vi "Test_ADC.vi"() -> ()   [LabVIEW 2012]
uses:
  STM32-CoreBD.lvlib
panel:
  out "Error":u32
  out "Error Out":errorcluster caption="错误输出"
  in  "停止":bool
  out "数值":i32
  out "波形图":waveform(dbl)(graph)
  in  "SampleRate":u32=250000 min=1000 max=250000 step=1000
  in  "Points(X*5k)":u8=1 min=1 max=100
  in  "Channel":enum16{"Channel A", "Channel B"}(ring)
  in  "VISA资源输入":refnum<visa-resource-name>
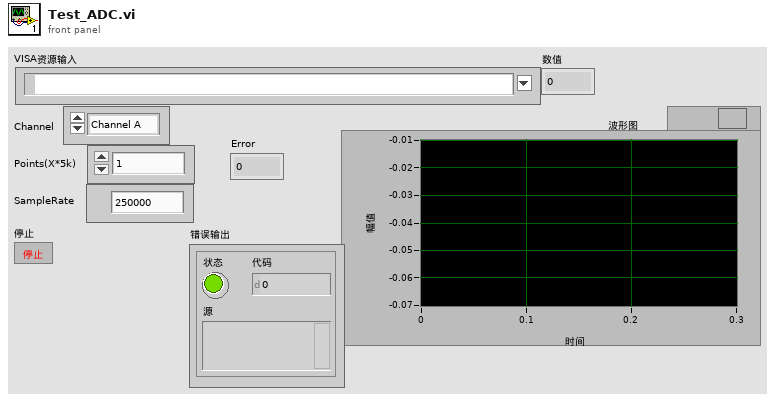
[diagram p1: front panel]
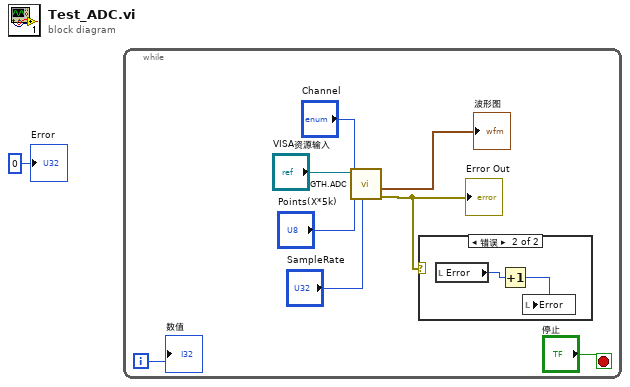
[diagram p0: block diagram]
diagram:
  n1 = while {
    i -> [w4]
    stop <- "停止" stop-if-true
    n2 = call "GTH.ADC.vi"("SampleRate"="SampleRate", "Points(X*5k)"="Points(X*5k)", "Channel"="Channel", "VISA资源输入"="VISA资源输入") -> ("Error Out"=w2:errorcluster, "波形图"=→"波形图":waveform(dbl))  [unwired: 4 in, 2 out]
    "Error Out" <- w2
    n3 = case shown="错误" w2 {
      frame No Error {
      }
      frame Error {
        n4 = local read "Error"() -> (w11:u32)
        n5 = Increment(x=w11) -> (x+1=w10:u32)
        n6 = local write "Error"(w10) -> ()
      }
    }
    "数值" <- w4
  }
  "Error" <- u32 0 ("Error")
